vi "Sequence Execution.vi"() -> ()   [LabVIEW 2013, in "Simple Sequence Tools - Execution.lvlib"]
uses:
  Simple Sequence Execution Tool Support.llb/Simple Sequence Tools - Execution.lvlib
  NationalInstruments.VeriStand.RealTimeSequenceDefinitionApi
  NationalInstruments.VeriStand.ClientAPI
  Simple Sequence Execution Tool Support.llb/NI_VS Workspace ExecutionAPI.lvlib
  Simple Sequence Execution Tool Support.llb/Simple Sequence Tools - Shared.lvlib
  Simple Sequence Execution Tool Support.llb/NI_VS Data Logging API.lvlib
panel:
  out "Total Iterations":u32=1 min=1 max=2
  out "Current Step":u32 min=1 max=5
  out "Current Iteration":u32=1 min=1 max=2
  in  "NIVS.Gateway IP Address":string="localhost"
  in  "NIVS.Workspace Event":refnum<event-registration>
  in  "Preview Mode":enum8{"Graph", "Table"}(ring)=enum."Table"
  in  "Start Step":u32 min=1 max=5
  in  "Start Iteration":u32=1 min=1 max=2
  in  "Log Channels":T1(ring)
  in  "Base File Name":string caption="Base File Name (timestamp included automatically)"
  in  "Enable Logging":bool
  in  "Abort":bool
  in  "Pause":bool
  in  "Start":bool
  in  "Profiles":string(combo)
  out "Graph":waveform(dbl)[](graph)
  out "Sequence":i32[](listbox)
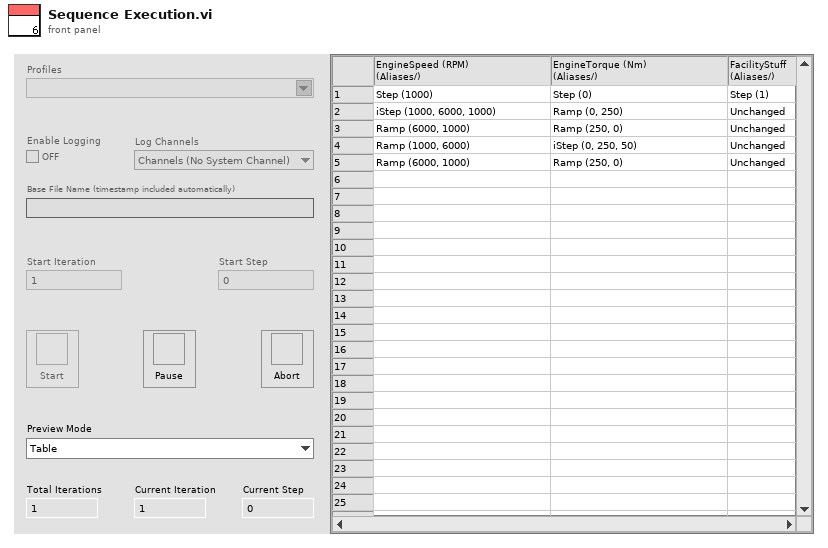
[diagram p1: front panel]
types:
  T1 = enum16{"Channels (No System Channel)", "Aliases", "All"}
  T2 = enum16{"Idle", "Initializing", "Running", "Paused", "Finalizing", "Complete"}
  T3 = cluster{"NIVS.BaseLogPath":path, "NIVS.SystemDefinitionFile":path, "NIVS.Events":cluster{"SequenceEvent":refnum<event-registration>, "SystemChangeEvent":refnum<event-registration>, "WorkspaceEvent":refnum<event-registration>}, "NIVS.SequenceState":enum16{"Idle", "Initializing", "Running", "Paused", "Finalizing", "Complete"}, "NIVS.GatewayIPAddress":string, "NIVS.DataLogSpecRef":refnum<k24>, "NIVS.DataLogManagerRef":refnum<k24>, "NIVS.LogSessionGUID":string, "NIVS.WorkspaceManager":refnum<k24>, "NIVS.Deployed":bool, "NIVS.ProfileRef":refnum<k24>, "NIVS.ProfileCallback":refnum<k27>, "NIVS.SystemStateRefs":cluster{"CustDatRef":refnum<user-event>, "EvtRef":refnum<k27>}, "UI.Abort":refnum<vi>, "UI.Pause":refnum<vi>, "UI.EnableLogging":refnum<vi>, "UI.Start":refnum<vi>, "UI.LogChannels":refnum<vi>, "UI.StartIteration":refnum<vi>, "UI.StartStep":refnum<vi>, "UI.Sequence":refnum<vi>, "UI.PreviewMode":refnum<vi>, "UI.Graph":refnum<vi>, "UI.BaseFileName":refnum<vi>, "UI.Profiles":refnum<vi>, "UI.CurrentStep":refnum<vi>, "UI.CurrentIteration":refnum<vi>, "UI.TotalIterations":refnum<vi>, "Sequence.AbortChannel":string, "Sequence.StepInfoChannel":string, "Sequence.Iterations":u32, "Sequence.IterationInfoChannel":string, "Sequence.#ofColumns":i32, "Events.State":refnum<user-event>, "Events.Test Result":refnum<user-event>, "Events.Progress":refnum<user-event>, "INI.Settings":cluster{"Build Location":path, "LoggingLocation":path}}
  T4 = enum8{"Enabled", "Disabled", "Disabled and Grayed Out"}
  T5 = cluster{"SequenceEvent":refnum<event-registration>, "SystemChangeEvent":refnum<event-registration>, "WorkspaceEvent":refnum<event-registration>}
  T6 = cluster{"Build Location":path, "LoggingLocation":path}
  T7 = cluster{"CustDatRef":refnum<user-event>, "EvtRef":refnum<k27>}
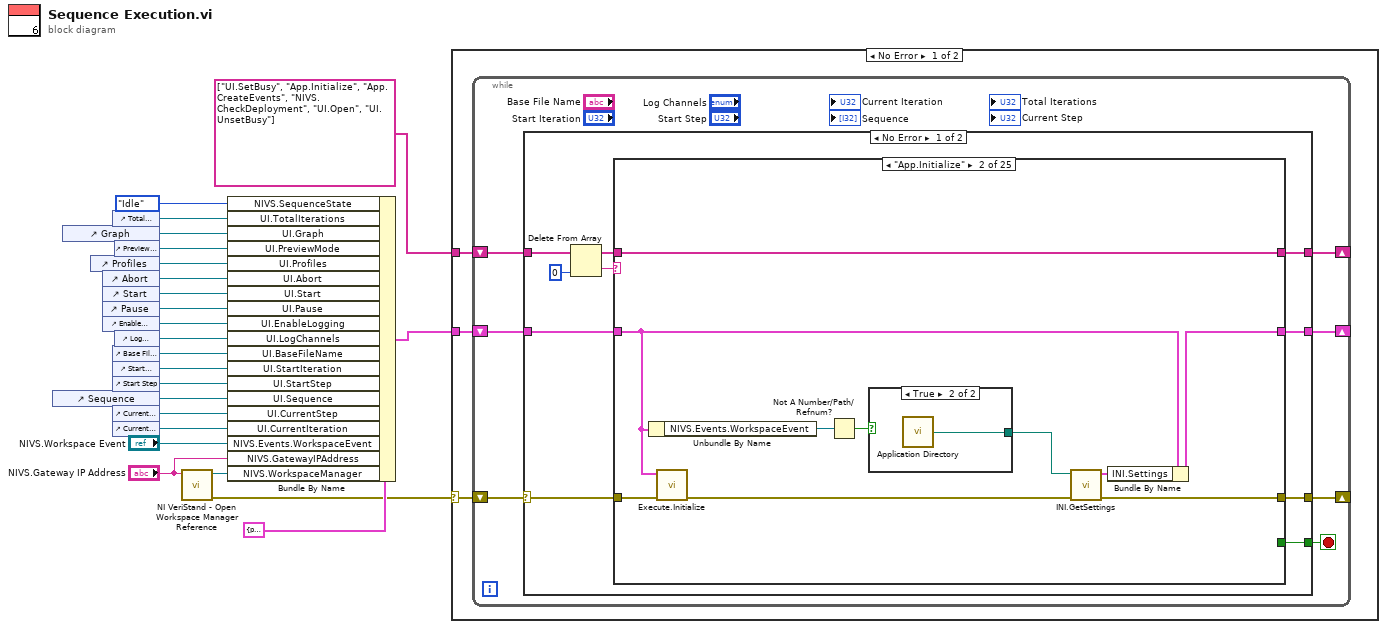
[diagram p0: block diagram]
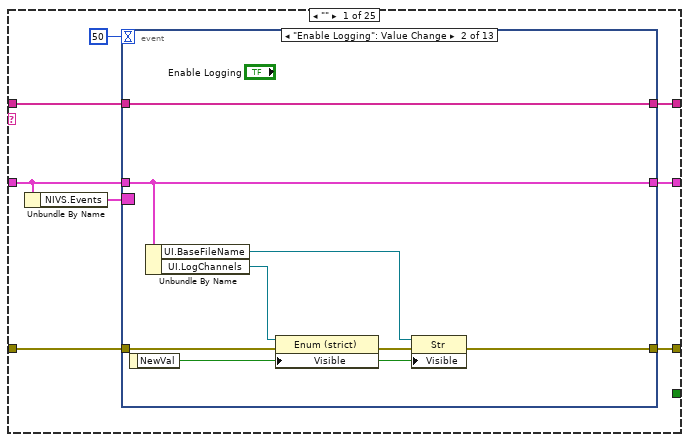
[diagram p2: hidden frame]
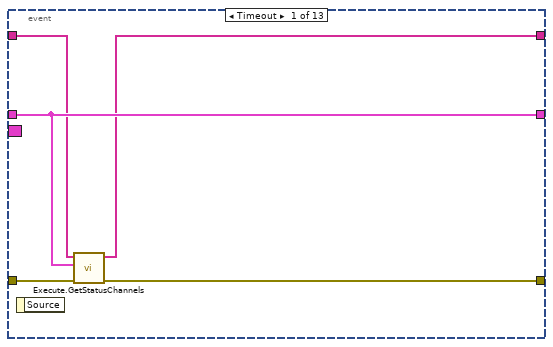
[diagram p3: hidden frame]
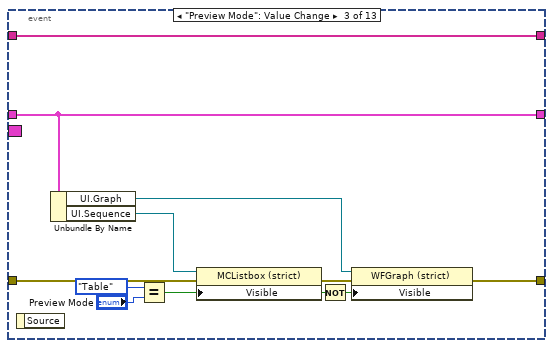
[diagram p4: hidden frame]
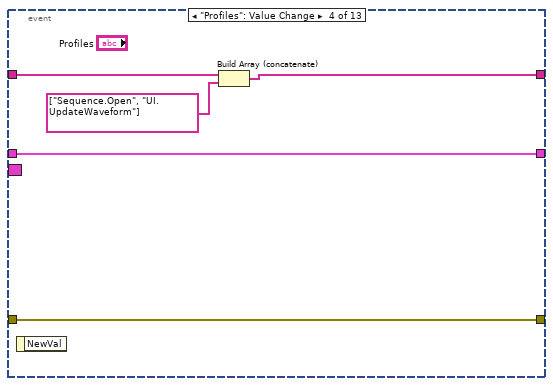
[diagram p5: hidden frame]
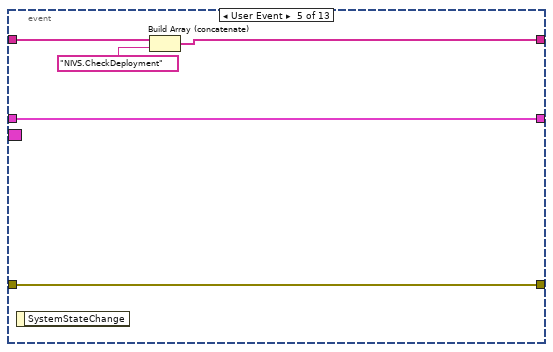
[diagram p6: hidden frame]
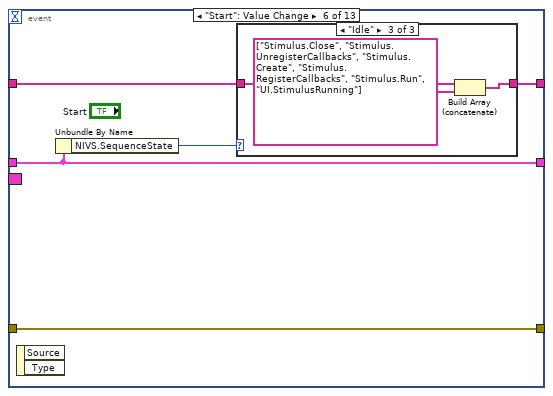
[diagram p7: hidden frame]
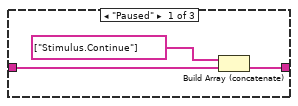
[diagram p8: hidden frame]
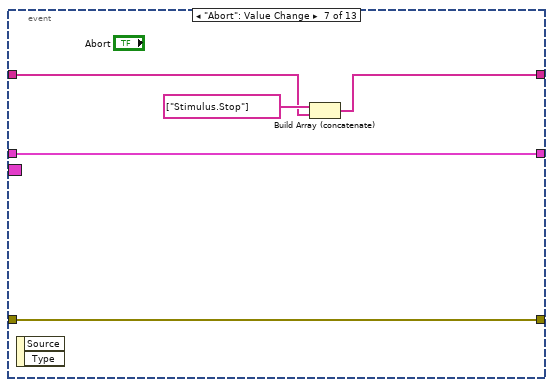
[diagram p10: hidden frame]
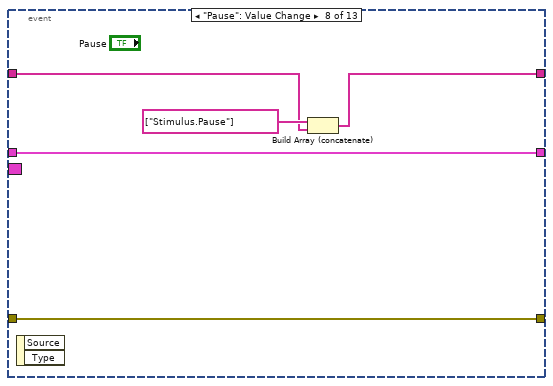
[diagram p11: hidden frame]
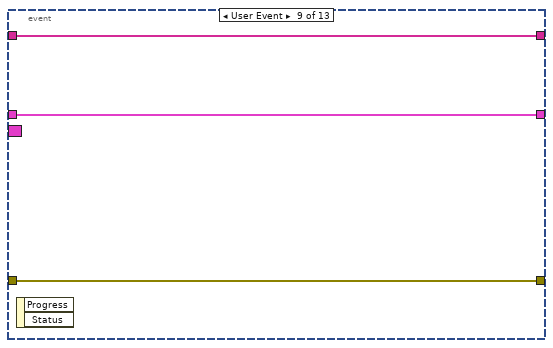
[diagram p12: hidden frame]
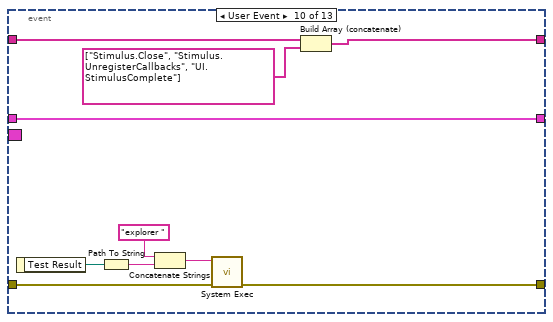
[diagram p13: hidden frame]
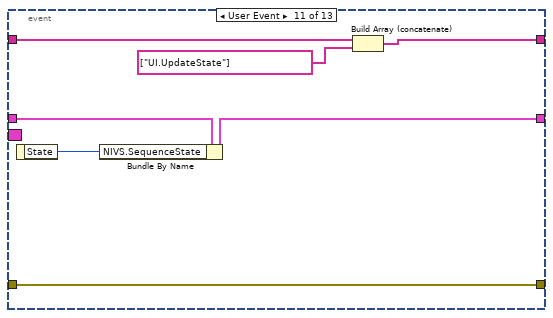
[diagram p14: hidden frame]
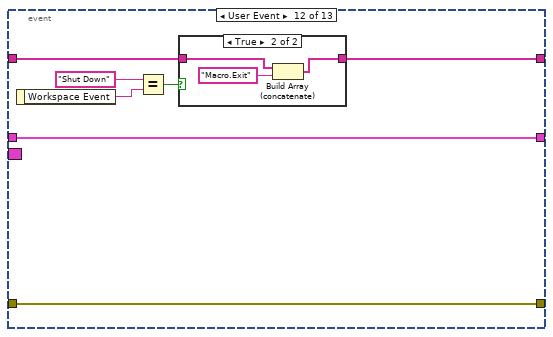
[diagram p15: hidden frame]
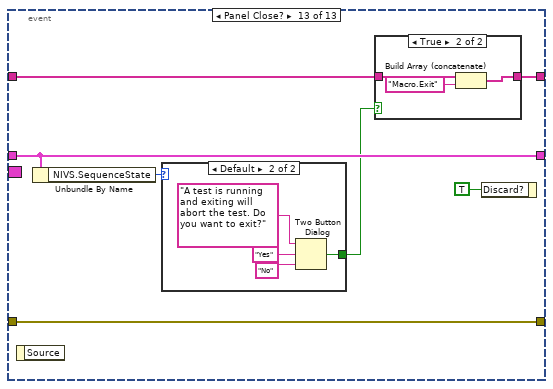
[diagram p17: hidden frame]
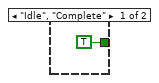
[diagram p19: hidden frame]
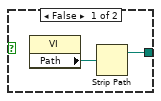
[diagram p20: hidden frame]
diagram:
  n1 = control-ref of="Sequence"() -> (w13:refnum<vi>)
  n2 = control-ref of="Graph"() -> (w22:refnum<vi>)
  n3 = control-ref of="Profiles"() -> (w11:refnum<vi>)
  n4 = control-ref of="Abort"() -> (w20:refnum<vi>)
  n5 = control-ref of="Start"() -> (w19:refnum<vi>)
  n6 = control-ref of="Pause"() -> (w18:refnum<vi>)
  n7 = control-ref of="Enable Logging"() -> (w17:refnum<vi>)
  n8 = control-ref of="Total Iterations"() -> (w4:refnum<vi>)
  n9 = control-ref of="Base File Name"() -> (w3:refnum<vi>)
  n10 = control-ref of="Start Iteration"() -> (w15:refnum<vi>)
  n11 = control-ref of="Start Step"() -> (w14:refnum<vi>)
  n12 = control-ref of="Current Step"() -> (w6:refnum<vi>)
  n13 = control-ref of="Current Iteration"() -> (w5:refnum<vi>)
  n14 = control-ref of="Preview Mode"() -> (w21:refnum<vi>)
  n15 = control-ref of="Log Channels"() -> (w16:refnum<vi>)
  n16 = call "NI VeriStand - Open Workspace Manager Reference.vi"("Gateway IP Address (\"\": localhost)"="NIVS.Gateway IP Address") -> ("error out"=w2:errorcluster, "WorkspaceManager"=w7:refnum<k24>)  [unwired: 9 in]
  n17 = Bundle By Name(cluster=T3 {"NIVS.BaseLogPath"=path "", "NIVS.SystemDefinitionFile"=path "", "NIVS.Events"={"SequenceEvent"=refnum, "SystemChangeEvent"=refnum, "WorkspaceEvent"=refnum}, "NIVS.SequenceState"=enum."Idle", "NIVS.GatewayIPAddress"="", "NIVS.DataLogSpecRef"=refnum, "NIVS.DataLogManagerRef"=refnum, "NIVS.LogSessionGUID"="", "NIVS.WorkspaceManager"=refnum, "NIVS.Deployed"=FALSE, "NIVS.ProfileRef"=refnum, "NIVS.ProfileCallback"=refnum, "NIVS.SystemStateRefs"={"CustDatRef"=refnum, "EvtRef"=refnum}, "UI.Abort"=refnum, "UI.Pause"=refnum, "UI.EnableLogging"=refnum, "UI.Start"=refnum, "UI.LogChannels"=refnum, "UI.StartIteration"=refnum, "UI.StartStep"=refnum, "UI.Sequence"=refnum, "UI.PreviewMode"=refnum, "UI.Graph"=refnum, "UI.BaseFileName"=refnum, "UI.Profiles"=refnum, "UI.CurrentStep"=refnum, "UI.CurrentIteration"=refnum, "UI.TotalIterations"=refnum, "Sequence.AbortChannel"="", "Sequence.StepInfoChannel"="", "Sequence.Iterations"=0, "Sequence.IterationInfoChannel"="", "Sequence.#ofColumns"=0, "Events.State"=refnum, "Events.Test Result"=refnum, "Events.Progress"=refnum, "INI.Settings"={"Build Location"=path "", "LoggingLocation"=path ""}} ("Cluster"), "NIVS.SequenceState"=T2."Idle", "UI.TotalIterations"=w4, "UI.Graph"=w22, "UI.PreviewMode"=w21, "UI.Profiles"=w11, "UI.Abort"=w20, "UI.Start"=w19, "UI.Pause"=w18, "UI.EnableLogging"=w17, "UI.LogChannels"=w16, "UI.BaseFileName"=w3, "UI.StartIteration"=w15, "UI.StartStep"=w14, "UI.Sequence"=w13, "UI.CurrentStep"=w6, "UI.CurrentIteration"=w5, "NIVS.Events.WorkspaceEvent"="NIVS.Workspace Event", "NIVS.GatewayIPAddress"="NIVS.Gateway IP Address", "NIVS.WorkspaceManager"=w7) -> (w12:T3)
  n18 = case shown="No Error" w2 {
    selector: w2 -> [w24 _]
    tunnel: string[] ["UI.SetBusy", "App.Initialize", "App.CreateEvents", "NIVS.CheckDeployment", "UI.Open", "UI.UnsetBusy"] -> [w26 _]
    tunnel: w12 -> [w25 w387]
    frame No Error {
      n19 = while {
        shift-right: [w32] -> _
        shift-left: w26 -> [w33]
        shift-right: [w30] -> _
        shift-left: w25 -> [w31]
        shift-right: [w28] -> _
        shift-left: w24 -> [w29]
        stop <- w27 stop-if-true
        n20 = case shown="No Error" w29 {
          selector: w29 -> [w34 w383]
          tunnel: w33 -> [w36 w386]
          tunnel: [w42 w386] -> w32
          tunnel: w31 -> [w40 w385]
          tunnel: [w39 w385] -> w30
          tunnel: [w38 w382] -> w28
          tunnel: [w37 _] -> w27
          frame No Error {
            n21 = Delete From Array(array=w36, index=0) -> (deleted portion=w43:string, array with subset deleted=w41:string[])  [unwired: 1 in]
            n22 = case shown="\"App.Initialize\"" w43 {
              tunnel: [w49 w159 w172 w176 w177 w186 w190 w199 w233 w238 w251 w256 w262 w272 w284 w301 w312 w316 w319 w322 w326 w330 w343 w359 w381] -> w42
              tunnel: w41 -> [w48 w159 w172 w176 w177 w186 w191 w200 w233 w238 w251 w256 w262 w272 w284 w301 w312 w316 w319 w322 w326 w330 w343 w359 w381]
              tunnel: w40 -> [w45 w158 w168 w173 w181 w187 w193 w202 w230 w235 w242 w253 w261 w271 w281 w303 w310 w315 w318 w321 w323 w327 w342 w353 w380]
              tunnel: [w51 w162 w170 w173 w181 w187 w193 w201 w229 w234 w243 w252 w261 w271 w281 w303 w310 w315 w318 w321 w323 w327 w342 w353 w380] -> w39
              tunnel: [w46 w163 w171 w174 w185 w189 w194 w197 w231 w236 w249 w255 w257 w267 w282 w300 w311 w313 w317 w320 w324 w328 w336 w357 w379] -> w38
              tunnel: w34 -> [w47 w164 w169 w175 w185 w189 w194 w198 w232 w237 w250 w254 w258 w268 w283 w300 w311 w314 w317 w320 w325 w329 w339 w358 w379]
              tunnel: [_ _ _ _ _ TRUE _ _ _ _ _ _ _ _ _ _ _ _ _ _ _ _ _ _ _] -> w37
              frame "" {
                n23 = Unbundle By Name(w45) -> ("NIVS.Events"=w44:T5)
                n24 = event shown="[1] \"Enable Logging\": Value Change" {
                  selector: w44 -> [_ _ _ _ _ _ _ _ _ _ _ _ _]
                  dyn-events: _ -> [_ _ _ _ _ _ _ _ _ _ _ _ _]
                  timeout: 50 -> [_ _ _ _ _ _ _ _ _ _ _ _ _]
                  tunnel: [w53 w64 w75 w79 w84 w88 w98 w103 w110 w118 w121 w129 w142] -> w49
                  tunnel: w48 -> [w54 w64 w75 w80 w85 w89 w99 w104 w110 w119 w122 w132 w145]
                  tunnel: [w56 w63 w72 w78 w82 w87 w102 w107 w109 w120 w124 w134 w141] -> w51
                  tunnel: w45 -> [w56 w63 w72 w78 w82 w87 w102 w107 w109 w120 w125 w134 w141]
                  tunnel: [w52 w57 w65 w77 w81 w90 w101 w106 w108 w115 w127 w133 w144] -> w46
                  tunnel: w47 -> [w55 w61 w66 w77 w81 w90 w101 w106 w108 w116 w127 w133 w144]
                  event Timeout {
                    n25 = event-data() -> ()  [unwired: 1 in, 1 out]
                    n26 = call "Execute.GetStatusChannels.vi"("error in (no error)"=w55, "Cluster"=w56, "Commands"=w54) -> ("error out"=w52:errorcluster, "Commands out"=w53:string[])  [unwired: 7 in]
                  }
                  event "Enable Logging": Value Change {
                    n27 = event-data() -> ("NewVal"=w58:bool)  [unwired: 1 in]
                    n28 = Unbundle By Name(w63) -> ("UI.BaseFileName"=w59:refnum<vi>, "UI.LogChannels"=w62:refnum<vi>)
                    n29 = property class="Enum (strict)"(reference=w62, error in=w61, "Visible"=w58) -> (error out=w60:errorcluster)  [unwired: 1 out]
                    n30 = property class="Str"(reference=w59, error in=w60, "Visible"=w58) -> (error out=w57:errorcluster)  [unwired: 1 out]
                  }
                  event "Preview Mode": Value Change {
                    n31 = event-data() -> ()  [unwired: 1 in, 1 out]
                    n32 = Unbundle By Name(w72) -> ("UI.Graph"=w70:refnum<vi>, "UI.Sequence"=w71:refnum<vi>)
                    n33 = Equal?(x=enum8{"Graph", "Table"}."Table" ("y"), y="Preview Mode") -> (x = y?=w68:bool)
                    n34 = property class="MCListbox (strict)"(reference=w71, error in=w66, "Visible"=w68) -> (error out=w69:errorcluster)  [unwired: 1 out]
                    n35 = Not(x=w68) -> (.not. x?=w67:bool)
                    n36 = property class="WFGraph (strict)"(reference=w70, error in=w69, "Visible"=w67) -> (error out=w65:errorcluster)  [unwired: 1 out]
                  }
                  event "Profiles": Value Change {
                    n37 = event-data() -> ()  [unwired: 1 in, 1 out]
                    n38 = Build Array (concatenate)(w80, string[] ["Sequence.Open", "UI.UpdateWaveform"]) -> (w79:string[])
                  }
                  event User Event {
                    n39 = event-data() -> ()  [unwired: 1 in, 1 out]
                    n40 = Build Array (concatenate)(w85, "NIVS.CheckDeployment") -> (w84:string[])
                  }
                  event "Start": Value Change {
                    n41 = event-data() -> ()  [unwired: 1 in, 2 out]
                    n42 = Unbundle By Name(w87) -> ("NIVS.SequenceState"=w86:T2)
                    n43 = case shown="\"Idle\"" w86 {
                      tunnel: w89 -> [w92 w94 w97]
                      tunnel: [w91 w94 w96] -> w88
                      frame "Paused" {
                        n44 = Build Array (concatenate)(string[] ["Stimulus.Continue"] ("array"), w92) -> (w91:string[])
                      }
                      frame Default {
                      }
                      frame "Idle" {
                        n45 = Build Array (concatenate)(w97, string[] ["Stimulus.Close", "Stimulus.UnregisterCallbacks", "Stimulus.Create", "Stimulus.RegisterCallbacks", "Stimulus.Run", "UI.StimulusRunning"] ("array")) -> (w96:string[])
                      }
                    }
                  }
                  event "Abort": Value Change {
                    n46 = event-data() -> ()  [unwired: 1 in, 2 out]
                    n47 = Build Array (concatenate)(string[] ["Stimulus.Stop"] ("array"), w99) -> (w98:string[])
                  }
                  event "Pause": Value Change {
                    n48 = event-data() -> ()  [unwired: 1 in, 2 out]
                    n49 = Build Array (concatenate)(string[] ["Stimulus.Pause"] ("array"), w104) -> (w103:string[])
                  }
                  event User Event {
                    n50 = event-data() -> ()  [unwired: 1 in, 2 out]
                  }
                  event User Event {
                    n51 = event-data() -> ("Test Result"=w114:path)  [unwired: 1 in]
                    n52 = Path To String(path=w114) -> (string=w113:string)
                    n53 = Concatenate Strings("explorer " ("string"), w113) -> (w112:string)
                    n54 = call "System Exec.vi"("error in (no error)"=w116, "command line"=w112) -> ("error out"=w115:errorcluster)  [unwired: 6 in, 3 out]
                    n55 = Build Array (concatenate)(w119, string[] ["Stimulus.Close", "Stimulus.UnregisterCallbacks", "UI.StimulusComplete"]) -> (w118:string[])
                  }
                  event User Event {
                    n56 = event-data() -> ("State"=w126:i32)  [unwired: 1 in]
                    n57 = Bundle By Name(cluster=w125, "NIVS.SequenceState"=w126) -> (w124:T3)
                    n58 = Build Array (concatenate)(w122, string[] ["UI.UpdateState"] ("array")) -> (w121:string[])
                  }
                  event User Event {
                    n59 = event-data() -> ("Workspace Event"=w128:string)  [unwired: 1 in]
                    n60 = Equal?(x="Shut Down" ("y"), y=w128) -> (x = y?=w130:bool)
                    n61 = case shown="True" w130 {
                      tunnel: w132 -> [w135 w138]
                      tunnel: [w135 w136] -> w129
                      frame False {
                      }
                      frame True {
                        n62 = Build Array (concatenate)(w138, "Macro.Exit" ("y")) -> (w136:string[])
                      }
                    }
                  }
                  event Panel Close? {
                    n63 = event-data() -> ()  [unwired: 1 in, 1 out]
                    n64 = Unbundle By Name(w141) -> ("NIVS.SequenceState"=w140:T2)
                    n65 = case shown="Default" w140 {
                      tunnel: [TRUE ("T button?") w151] -> w139
                      frame "Idle", "Complete" {
                      }
                      frame Default {
                        n66 = Two Button Dialog(message="A test is running and exiting will abort the test. Do you want to exit?", 1:"No" ("F button name (\"Cancel\")"), 2:"Yes" ("T button name (\"OK\")")) -> (T button?=w151:bool)
                      }
                    }
                    n67 = case shown="True" w139 {
                      tunnel: w145 -> [w146 w149]
                      tunnel: [w146 w148] -> w142
                      frame False {
                      }
                      frame True {
                        n68 = Build Array (concatenate)(w149, "Macro.Exit") -> (w148:string[])
                      }
                    }
                    n69 = event-data("Discard?"=TRUE) -> ()  [unwired: 1 in, 1 out]
                  }
                }
              }
              frame "App.Initialize" {
                n70 = Unbundle By Name(w158) -> ("NIVS.Events.WorkspaceEvent"=w157:refnum<event-registration>)
                n71 = call "Execute.Initialize.vi"("error in (no error)"=w164, "Cluster"=w158) -> ("error out"=w160:errorcluster)  [unwired: 9 in]
                n72 = Not A Number/Path/Refnum?(number/path/refnum=w157) -> (NaN/Path/Refnum?=w155:bool)
                n73 = case shown="True" w155 {
                  tunnel: [w165 w167] -> w156
                  frame False {
                    n74 = property class="VI"() -> ("Path"=w166:path)  [unwired: 2 in, 2 out]
                    n75 = Strip Path(path=w166) -> (stripped path=w165:path)  [unwired: 1 out]
                  }
                  frame True {
                    n76 = call "Application Directory.vi"() -> ("Application Directory"=w167:path)
                  }
                }
                n77 = call "INI.GetSettings.vi"("error in (no error)"=w160, "INI Folder Location"=w156) -> ("error out"=w163:errorcluster, "INI.Settings"=w161:T6)  [unwired: 8 in]
                n78 = Bundle By Name(cluster=w158, "INI.Settings"=w161) -> (w162:T3)
              }
              frame "App.CreateEvents" {
                n79 = call "Execute.CreateEvents.vi"("error in (no error)"=w169, "Cluster in"=w168) -> ("error out"=w171:errorcluster, "Cluster out"=w170:T3)  [unwired: 8 in]
              }
              frame "App.LoadSequences" {
                n80 = call "Execute.LoadSequences.vi"("error in (no error)"=w175, "Cluster"=w173) -> ("error out"=w174:errorcluster)  [unwired: 9 in]
              }
              frame "App.CloseReferences" {
                n81 = Unbundle By Name(w181) -> ("Events.State"=w182:refnum<user-event>, "Events.Test Result"=w183:refnum<user-event>, "Events.Progress"=w184:refnum<user-event>, "NIVS.Events"=w180:T5, "NIVS.SystemStateRefs"=w179:T7, "NIVS.WorkspaceManager"=w178:refnum<k24>)
                n82 = call "NI VeriStand - Close Workspace Manager Reference.vi"("WorkspaceManager"=w178) -> ()  [unwired: 10 in, 1 out]
                n83 = call "NI VeriStand - Close Engine State Change Notification.vi"("SystemStateRefs"=w179) -> ()  [unwired: 10 in, 1 out]
                n84 = Unregister For Events(event registration refnum=w180) -> ()  [unwired: 1 in, 1 out]
                n85 = Destroy User Event(user event=w184) -> ()  [unwired: 1 in, 1 out]
                n86 = Destroy User Event(user event=w183) -> ()  [unwired: 1 in, 1 out]
                n87 = Destroy User Event(user event=w182) -> ()  [unwired: 1 in, 1 out]
                n88 = disable-structure shown="Enabled" {
                  frame Enabled {
                    n89 = invoke class="VI" method="FP.Close"() -> ()  [unwired: 3 in, 3 out]
                  }
                  frame Disabled {
                  }
                }
              }
              frame "App.Exit" {
              }
              frame "Macro.Exit" {
                n90 = Build Array (concatenate)(w191, string[] ["Stimulus.Stop", "Stimulus.Close", "Stimulus.UnregisterCallbacks", "App.CloseReferences", "App.Exit"]) -> (w190:string[])
              }
              frame "NIVS.CheckDeployment" {
                n91 = Unbundle By Name(w202) -> ("INI.Settings.LoggingLocation"=w196:path, "NIVS.WorkspaceManager"=w203:refnum<k24>)
                n92 = call "NI VeriStand - Get System State.vi"("error in (no error)"=w198, "WorkspaceManager in"=w203) -> ("error out"=w197:errorcluster, "System State"=w204:u8, "System Definition File"=w195:path)  [unwired: 5 in, 2 out]
                n93 = case shown="1" w204 {
                  tunnel: w200 -> [w208 w222]
                  tunnel: [w207 w221] -> w199
                  tunnel: w202 -> [w211 w219]
                  tunnel: [w210 w217] -> w201
                  tunnel: w196 -> [_ w214]
                  tunnel: w195 -> [_ w213]
                  frame 0, Default {
                    w205 = path ""
                    # "Not connected"
                    n94 = Bundle By Name(cluster=w211, "NIVS.Deployed"=FALSE ("Connected"), "NIVS.SystemDefinitionFile"=w205, "NIVS.BaseLogPath"=w205) -> (w210:T3)
                    n95 = Build Array (concatenate)(w208, "App.Initialize") -> (w207:string[])
                  }
                  frame 1 {
                    # "Connected"
                    n96 = Empty String/Path?(string/path=w214) -> (empty?=w215:bool)
                    n97 = case shown="True" w215 {
                      tunnel: [w224 w226] -> w216
                      tunnel: w214 -> [w224 _]
                      tunnel: w213 -> [w223 w225]
                      tunnel: [w223 w225] -> w212
                      frame False {
                      }
                      frame True {
                        n98 = Strip Path(path=w225) -> (stripped path=w228:path)  [unwired: 1 out]
                        n99 = Build Path(base path=w228, name or relative path="Logs") -> (appended path=w226:path)
                      }
                    }
                    n100 = Build Array (concatenate)(string[] ["App.LoadSequences", "UI.Connected"], w222) -> (w221:string[])
                    n101 = Bundle By Name(cluster=w219, "NIVS.Deployed"=TRUE ("Connected"), "NIVS.BaseLogPath"=w216, "NIVS.SystemDefinitionFile"=w212) -> (w217:T3)
                  }
                }
              }
              frame "Sequence.Open" {
                n102 = call "Execute.InitializeSequence.vi"("error in (no error)"=w232, "State Variables"=w230) -> ("error out"=w231:errorcluster, "State Variables"=w229:T3)  [unwired: 8 in]
              }
              frame "Stimulus.Create" {
                n103 = call "Execute.RunStimulus.vi"("error in (no error)"=w237, "State Variables"=w235) -> ("error out"=w236:errorcluster, "State Variables"=w234:T3)  [unwired: 8 in]
              }
              frame "Stimulus.RegisterCallbacks" {
                n104 = Unbundle By Name(w242) -> ("NIVS.ProfileRef"=w248:refnum<k24>, "Events.Progress"=w247:refnum<user-event>, "Events.Test Result"=w246:refnum<user-event>, "Events.State"=w245:refnum<user-event>)
                n105 = vi-ref "SequenceEvent.ProgressChanged.vi"() -> ("vi reference"=w241:refnum<vi>)
                n106 = vi-ref "SequenceEvent.ExecuteCompleted.vi"() -> ("vi reference"=w240:refnum<vi>)
                n107 = vi-ref "SequenceEvent.PropertyChanged.vi"() -> ("vi reference"=w239:refnum<vi>)
                n108 = node(w250, w248, w241, w247, w248, w240, w246, w248, w239, w245) -> (w244:refnum<k27>, w249:errorcluster)  [unwired: 1 in]
                n109 = Bundle By Name(cluster=w242, "NIVS.ProfileCallback"=w244) -> (w243:T3)
              }
              frame "Stimulus.Run" {
                n110 = call "Execute.Stimulus.Run.vi"("error in (no error)"=w254, "Cluster in"=w253) -> ("error out"=w255:errorcluster, "Cluster out"=w252:T3)  [unwired: 8 in]
              }
              frame "Stimulus.Pause" {
                n111 = Unbundle By Name(w261) -> ("NIVS.SequenceState"=w259:T2, "NIVS.ProfileRef"=w260:refnum<k24>)
                n112 = case shown="\"Running\"" w259 {
                  tunnel: w260 -> [_ w266]
                  tunnel: w258 -> [w263 w265]
                  tunnel: [w263 w264] -> w257
                  frame "Idle", Default {
                  }
                  frame "Running" {
                    n113 = invoke class="StimulusProfile" method="Pause"(reference=w266, error in=w265) -> (error out=w264:errorcluster)  [unwired: 1 in, 2 out]
                  }
                }
              }
              frame "Stimulus.Continue" {
                n114 = Unbundle By Name(w271) -> ("NIVS.SequenceState"=w270:T2, "NIVS.ProfileRef"=w269:refnum<k24>)
                n115 = case shown="\"Paused\"" w270 {
                  tunnel: w269 -> [_ w276]
                  tunnel: w268 -> [w273 w275]
                  tunnel: [w273 w274] -> w267
                  frame "Idle", Default {
                  }
                  frame "Paused" {
                    n116 = invoke class="StimulusProfile" method="Continue"(reference=w276, error in=w275) -> (error out=w274:errorcluster)  [unwired: 1 in, 2 out]
                  }
                }
              }
              frame "Stimulus.Stop" {
                n117 = Unbundle By Name(w281) -> ("NIVS.WorkspaceManager"=w277:refnum<k24>, "Sequence.AbortChannel"=w278:string, "NIVS.SequenceState"=w279:T2, "NIVS.ProfileRef"=w280:refnum<k24>)
                n118 = case shown="\"Running\", \"Paused\", Default" w279 {
                  tunnel: w280 -> [_ w287]
                  tunnel: w283 -> [w285 w291]
                  tunnel: [w285 w286] -> w282
                  tunnel: w278 -> [_ w290]
                  tunnel: w277 -> [_ w289]
                  frame "Idle" {
                  }
                  frame "Running", "Paused", Default {
                    n119 = case shown="Default" w290 {
                      selector: w290 -> [_ w294]
                      tunnel: w291 -> [w292 w297]
                      tunnel: [w292 w296] -> w288
                      tunnel: w289 -> [_ w295]
                      frame "" {
                      }
                      frame Default {
                        n120 = call "NI VeriStand - Set Single Channel Value.vi"("error in (no error)"=w297, "Value"=1.0, "Channel"=w294, "WorkspaceManager in"=w295) -> ("error out"=w296:errorcluster)  [unwired: 6 in, 1 out]
                      }
                    }
                    n121 = invoke class="StimulusProfile" method="Stop"(reference=w287, error in=w288) -> (error out=w286:errorcluster)  [unwired: 1 in, 2 out]
                  }
                }
              }
              frame "Stimulus.Close" {
                n122 = Unbundle By Name(w303) -> ("NIVS.ProfileRef"=w302:refnum<k24>, "NIVS.DataLogManagerRef"=w299:refnum<k24>, "NIVS.LogSessionGUID"=w298:string)
                n123 = case shown="Default" w298 {
                  selector: w298 -> [_ w305]
                  tunnel: w299 -> [_ w308]
                  tunnel: [_ w304] -> _
                  frame "" {
                  }
                  frame Default {
                    n124 = call "Stop Data Logging Session.vi"("Session Name in"=w305, "Data Logging Manager Ref in"=w308) -> ("error out"=w306:errorcluster, "Data Logging Manager Ref out"=w307:refnum<k24>)  [unwired: 7 in, 1 out]
                    n125 = call "Close Data Logging Manager Reference.vi"("error in (no error)"=w306, "Data Logging Manager Ref in"=w307) -> ("error out"=w304:errorcluster)  [unwired: 9 in]
                  }
                }
                n126 = Close Reference(reference=w302) -> ()  [unwired: 1 in, 1 out]
              }
              frame "Stimulus.UnregisterCallbacks" {
                n127 = Unbundle By Name(w310) -> ("NIVS.ProfileCallback"=w309:refnum<k27>)
                n128 = Unregister For Events(event registration refnum=w309) -> ()  [unwired: 1 in, 1 out]
              }
              frame "UI.Open" {
                n129 = invoke class="VI" method="FP.Open"(error in=w314) -> (error out=w313:errorcluster)  [unwired: 4 in, 4 out]
              }
              frame "UI.SetBusy" {
                n130 = call "Set Busy.vi"() -> ()  [unwired: 10 in, 2 out]
              }
              frame "UI.UnsetBusy" {
                n131 = call "Unset Busy.vi"() -> ()  [unwired: 11 in, 1 out]
              }
              frame "UI.StimulusComplete" {
                n132 = call "Execute.UI.Complete.vi"("error in (no error)"=w325, "Cluster"=w323) -> ("error out"=w324:errorcluster)  [unwired: 9 in]
              }
              frame "UI.StimulusRunning" {
                n133 = call "Execute.UI.Running.vi"("error in (no error)"=w329, "Cluster"=w327) -> ("error out"=w328:errorcluster)  [unwired: 9 in]
              }
              frame "UI.UpdateState" {
                n134 = Unbundle By Name(w342) -> ("UI.Start"=w332:refnum<vi>, "UI.Abort"=w333:refnum<vi>, "UI.Pause"=w340:refnum<vi>, "NIVS.SequenceState"=w341:T2)
                n135 = case shown="\"Paused\"" w341 {
                  tunnel: [w345 w346 T4."Disabled and Grayed Out" ("Disabled") w350] -> w335
                  tunnel: [T4."Disabled and Grayed Out" ("Disabled") w346 w347 T4."Enabled" ("f")] -> w331
                  tunnel: [w345 w346 w347 w350] -> w334
                  frame "Running" {
                    w345 = T4."Enabled" ("Disabled")
                  }
                  frame Default {
                    w346 = T4."Disabled and Grayed Out" ("Disabled")
                  }
                  frame "Paused" {
                    w347 = T4."Enabled" ("Disabled")
                  }
                  frame "Idle" {
                    w350 = T4."Disabled and Grayed Out" ("Disabled")
                  }
                }
                n136 = property class="Bool"(reference=w340, error in=w339, "DisabledEnum"=w335) -> (error out=w338:errorcluster)  [unwired: 1 out]
                n137 = property class="Bool"(reference=w333, error in=w338, "DisabledEnum"=w334) -> (error out=w337:errorcluster)  [unwired: 1 out]
                n138 = property class="Bool"(reference=w332, error in=w337, "DisabledEnum"=w331) -> (error out=w336:errorcluster)  [unwired: 1 out]
              }
              frame "UI.UpdateWaveform" {
                n139 = Unbundle By Name(w353) -> ("NIVS.SequenceState"=w352:T2, "UI.Graph"=w354:refnum<vi>, "UI.Sequence"=w355:refnum<vi>, "Sequence.#ofColumns"=w356:i32)
                n140 = case shown="Default" w352 {
                  tunnel: w358 -> [w366 w373]
                  tunnel: [w365 w378] -> w357
                  tunnel: w356 -> [w363 w376]
                  tunnel: w355 -> [w362 w368]
                  tunnel: w354 -> [w361 w375]
                  tunnel: [w360 w374] -> w351
                  frame "Idle" {
                    n141 = call "Sequence.BuildPreviewWaveform.vi"("WaveformGraph in"=w361, "error in (no error)"=w366, "Rows"=cluster{"Start Index":i32, "Length":i32} {"Start Index"=0, "Length"=-1}, "UI.Sequence#ofColumns"=w363, "SequenceRef"=w362) -> ("error out"=w365:errorcluster, "Wavefrom"=w360:waveform(dbl)[])  [unwired: 5 in]
                  }
                  frame Default {
                    n142 = property class="MCListbox (strict)"(reference=w368, error in=w373) -> (reference out=w367:refnum<vi>, error out=w372:errorcluster, "Value"=w370:i32[])
                    n143 = Index Array(array=w370) -> (element=w369:i32)  [unwired: 1 in]
                    n144 = Bundle By Name(cluster=cluster{"Start Index":i32, "Length":i32} {"Start Index"=0, "Length"=1} ("Rows"), "Start Index"=w369) -> (w371:cluster{"Start Index":i32, "Length":i32})
                    n145 = call "Sequence.BuildPreviewWaveform.vi"("WaveformGraph in"=w375, "error in (no error)"=w372, "Rows"=w371, "UI.Sequence#ofColumns"=w376, "SequenceRef"=w367) -> ("error out"=w378:errorcluster, "Wavefrom"=w374:waveform(dbl)[])  [unwired: 5 in]
                  }
                }
                "Graph" <- w351
              }
              frame Default {
              }
            }
          }
          frame Error {
            n146 = call "Simple Error Handler.vi"("error in (no error)"=w383) -> ("error out"=w384:errorcluster)  [unwired: 4 in, 4 out]
            n147 = call "Clear Errors.vi"("error in (no error)"=w384) -> ("error out"=w382:errorcluster)  [unwired: 6 in]
          }
        }
      }
    }
    frame Error {
      n148 = Unbundle By Name(w387) -> ("NIVS.Events.WorkspaceEvent"=w389:refnum<event-registration>)
      n149 = Not A Number/Path/Refnum?(number/path/refnum=w389) -> (NaN/Path/Refnum?=w388:bool)
      n150 = case shown="False" w388 {
        frame False {
          n151 = invoke class="VI" method="FP.Close"() -> ()  [unwired: 3 in, 3 out]
        }
        frame True {
        }
      }
      n152 = One Button Dialog(message="NI VeriStand is not open. Please open NI VeriStand before running this utility.") -> ()  [unwired: 1 in, 1 out]
    }
  }
